vi "Move From Output to Export Dir.vi"(0 "NI Build Specification in":refnum<class "Executable_LV.lvclass">, 11 "error IO":errorcluster) -> (4 "NI Build Specification out":refnum<class "Executable_LV.lvclass">, 15 "error out":errorcluster)   [LabVIEW 2017, in "CL_G3_VIComponentBuilder.lvlib" / "Executable_LV.lvclass"]
doc: "Moves the executable from the to a new folder in the Component's export directory. The new folder is named after the executables build spec name."
uses:
  Executable_LV.lvclass
  C:/Tool Chain Support/Software Module Builder/Source/Exports/NI Build Specification_LV/NI Build Specification_LV.lvclass
  C:/Tool Chain Support/Software Module Builder/Source/Exports/Exports/Export.lvclass
  <vilib>/AppBuilder/AB_API/common/AB_API Build Object Selector.ctl
  NI Build Specification_LV/NI Build Specification_LV.lvclass/NI Build Specification_LV.ctl
  Exports/Export.lvclass/Export.ctl
  NI Build Specification_LV/Accessors/Read TargetRef Containting Build Spec.vi
  NI Build Specification_LV/Accessors/Read Project Reference.vi
  Exports/Accessors/Read Component Export Dir.vi
  NI Build Specification_LV/Accessors/Read Export's Build Spec Name.vi
  Exports/Accessors/Write Built Export's Full Path.vi
  <vilib>/Utility/file.llb/Is Path and Not Empty.vi
  <vilib>/Utility/libraryn.llb/Check if File or Folder Exists.vi
  <vilib>/Utility/error.llb/Error Cluster From Error Code.vi
  <vilib>/AppBuilder/AB_API/Build/NI_AB_API_Build.lvclass
  NI Build Specification_LV/NI Build Specification_LV.lvclass
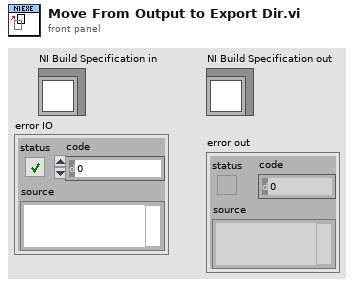
[diagram p1: front panel]
types:
  T1 = typedef "AB_API Build Object Selector.ctl" = enum16{"Source Distribution", "Deployable Source Distribution", "DLL", "EXE", "Packed Library", "Deployable Packed Library", "RT EXE", ".NET Interop Assembly"}
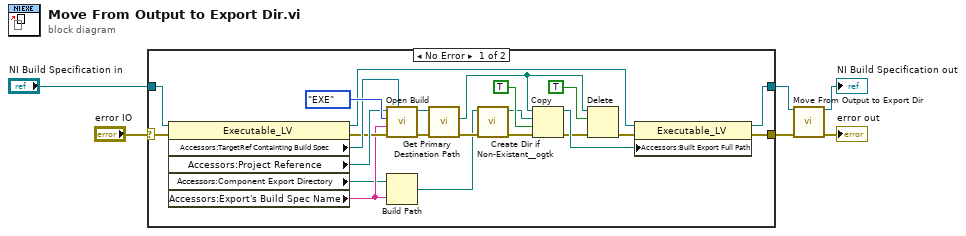
[diagram p0: block diagram]
diagram:
  n1 = case shown="No Error" "error IO" {
    selector: "error IO" -> [w14 w30]
    tunnel: "NI Build Specification in" -> [w27 w31]
    tunnel: [w26 w31] -> w6
    tunnel: [w21 w30] -> w3
    frame No Error {
      n2 = property class="Executable_LV"(reference=w27, error in=w14) -> (reference out=w25:refnum<class "Executable_LV.lvclass">, error out=w15:errorcluster, "Accessors:TargetRef Containting Build Spec"=w19:refnum<vi>, "Accessors:Project Reference"=w24:refnum<vi>, "Accessors:Component Export Directory"=w11:path, "Accessors:Export's Build Spec Name"=w12:string)
      n3 = call <vilib>:"Open Build.vi"("TargetItem Refnum"=w19, "error in (no error)"=w15, "Build specification name"=w12, "Build object selector"=AB_API_Build_Object_Selector."EXE", "Project Refnum"=w24) -> ("error out"=w23:errorcluster, "NI_AB_API_Build out"=w29:refnum<class "NI_AB_API_Build.lvclass">)  [unwired: 5 in]
      n4 = Build Path(base path=w11, name or relative path=w12) -> (appended path=w7:path)
      n5 = call-dynamic "Get Primary Destination Path.vi"("error in (no error)"=w23, "NI_AB_API_Build in"=w29) -> ("error out"=w10:errorcluster, "Primary destination path"=w16:path)  [unwired: 7 in, 1 out]
      n6 = call <userlib>:"Create Dir if Non-Existant__ogtk.vi"("error in (no error)"=w10, "Directory Path"=w7) -> ("error out"=w9:errorcluster, "dup Directory Path"=w8:path)  [unwired: 7 in, 1 out]
      n7 = Copy(8:w9, 9:TRUE ("overwrite (F)"), 10:w8, 11:w16) -> (0:w18:errorcluster, 3:w22:path)  [unwired: 1 in, 1 out]
      n8 = Delete(path (use dialog)=w16, entire hierarchy (F)=TRUE, error in=w18) -> (error out=w13:errorcluster)  [unwired: 2 in, 2 out]
      n9 = property class="Executable_LV"(reference=w25, error in=w13, "Accessors:Built Export Full Path"=w22) -> (reference out=w26:refnum<class "Executable_LV.lvclass">, error out=w21:errorcluster)
    }
    frame Error {
    }
  }
  n10 = call-parent "Move From Output to Export Dir.vi"("NI Build Specification in"=w6, "error IO"=w3) -> ("NI Build Specification out"=→"NI Build Specification out":refnum<class "Executable_LV.lvclass">, "error out"=→"error out":errorcluster)  [unwired: 12 in]
